vi "Receive Tree Item Close Event.vi"(8 "error in (no error)":errorcluster, 10 "TreeItemCloseMsg":refnum<class "TreeItemCloseMsg.lvclass">, 11 "IEventAggregator In":refnum<class "IEventAggregator.lvclass">) -> (0 "error out":errorcluster, 3 "IEventAggregator Out":refnum<class "IEventAggregator.lvclass">)   [LabVIEW 2020, in "MVA Framework.lvlib" / "ActorEvents.lvlib" / "IEventAggregator.lvclass"]
doc: "接收树形项关闭事件"
uses:
  IEventAggregator.lvclass
  IEventAggregator Messages/TreeItemCloseMsg/TreeItemCloseMsg.lvclass
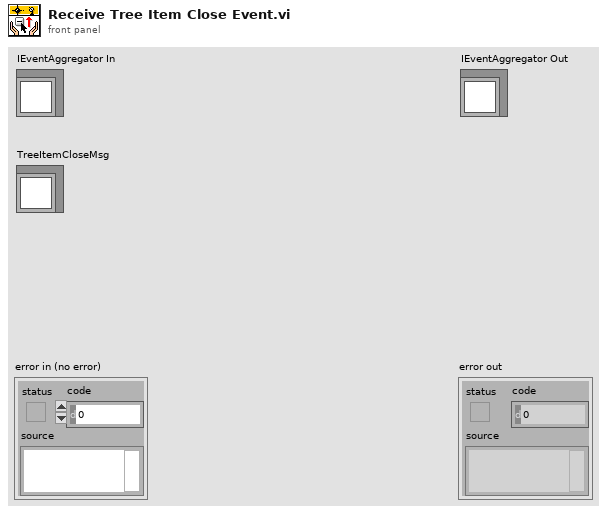
[diagram p1: front panel]
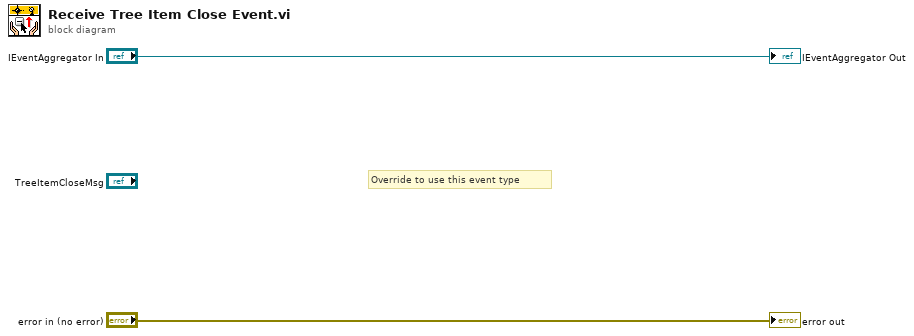
[diagram p0: block diagram]
diagram:
  # "Override to use this event type"
  "error out" <- "error in (no error)"
  "IEventAggregator Out" <- "IEventAggregator In"
